vi "main.vi"() -> ()   [LabVIEW 2011]
uses:
  <vilib>/Simulation/Scripting/Companion Diagram/SimConfigNode/SimParams.ctl
  <vilib>/Simulation/Scripting/Companion Diagram/SimConfigNode/_simSolvers.ctl
  <vilib>/Simulation/Implementation/Shared/SIMSCR Execution Mode.ctl
  <vilib>/Simulation/Param Hierarchy/Typedefs/SIMPH Param Control Actions.ctl
  <vilib>/Simulation/Implementation/Shared/NILVSim_FinalizeModel.vi
  <vilib>/Simulation/Utility/Implementation/SIM Halt.vi
  <vilib>/Simulation/SignalDisplay/Implementation/NILVSim Time Waveform.llb/SIM Time Waveform (scalar).vi
  <vilib>/Simulation/DataSources/Implementation/NILVSim Step.llb/SIM Step (scalar).vi
  <vilib>/Simulation/DataSources/Implementation/NILVSim Pulse Generator.llb/SIM Pulse Generator (scalar).vi
  <vilib>/Simulation/DataSources/Implementation/NILVSim Ramp.llb/SIM Ramp (scalar).vi
  <vilib>/Simulation/DataSources/Implementation/NILVSim Sine Wave.llb/SIM Sine Wave (scalar).vi
  <vilib>/Simulation/DataSources/Implementation/NILVSim Chirp Signal.llb/SIM Chirp Signal (scalar).vi
  <vilib>/Simulation/ContinuousLinear/Implementation/NILVSim Transfer Function.llb/SIM Transfer Function Collector (SISO).vi
  <vilib>/Simulation/ContinuousLinear/Implementation/NILVSim Transfer Function.llb/SIM Transfer Function Distributor (SISO CD).vi
  <vilib>/Simulation/Implementation/Shared/SIM Is Init or Final Stage.vi
  <vilib>/Simulation/Implementation/Shared/NILVSim_Manager.vi
  <vilib>/Simulation/Implementation/Shared/NILVSim_ParamChanged.vi
  <vilib>/Simulation/Utility/Implementation/NILVSim Get Time and IsAcceptedStep.vi
  <vilib>/Simulation/Implementation/Shared/SIM Unbundle Sim Info.vi
  <vilib>/Simulation/Implementation/Shared/NILVSim_GetModelError.vi
  <vilib>/Simulation/Implementation/Shared/SIM Bundle Sim Info.vi
  <vilib>/Simulation/Implementation/Shared/NILVSim_Initialize.vi
  <vilib>/addons/Control Design/_Model Construction/Model Creation.llb/CD Construct Transfer Function Model.vi
  <vilib>/addons/Control Design/_Model Construction/Model Creation.llb/Model Creation SubVI/cd_Create Transfer Function Model.vi
  <vilib>/addons/Control Design/_Frequency Response Analysis/Frequency Response.llb/Frequency Response subVI/cd_Bode (Transfer Function).vi
  <vilib>/addons/Control Design/_Frequency Response Analysis/Frequency Response.llb/Frequency Response subVI/cd_Nyquist (Transfer Function).vi
  <vilib>/addons/Control Design/_Dynamic Analysis/Dynamic Analysis.llb/Dynamic Analysis subVI/cd_Root Locus (Transfer Function).vi
  <vilib>/Simulation/Scripting/Companion Diagram/SimConfigNode/SimDog.xnode
  <vilib>/Simulation/Implementation/XNodeFramework/SimXNode/SimX.xnode
  <vilib>/addons/Control Design/_Model Construction/NI_LinSys_Model Creation.lvlib
  <vilib>/addons/Control Design/_Model Construction/Model Typedefs.llb/CD General Elements.ctl
  <vilib>/addons/Control Design/_Model Construction/NI_LinSys_Model Typedefs.lvlib
  <vilib>/addons/Control Design/_Model Construction/Model Typedefs.llb/CD Transfer Function Model (SISO).ctl
  <vilib>/addons/Control Design/_Model Construction/Model Typedefs.llb/CD Transfer Function Model (MIMO).ctl
  <vilib>/Simulation/ContinuousLinear/Implementation/NILVSim Transfer Function.llb/SIM Transfer Function (SISO CD).vi
  <vilib>/addons/Control Design/_Frequency Response Analysis/NI_CD_Frequency Response.lvlib
  <vilib>/addons/Control Design/_Dynamic Analysis/NI_CD_Dynamic Analysis.lvlib
  <vilib>/Simulation/Implementation/Shared/NI_SIM_Implementation.lvlib
panel:
  in  "Tab In-Disp":enum32{""}(tab)
  out "Signal In":waveform(dbl)(graph)={"t0"=timestamp(9343.2 s since 1904-01-01), "dt"=1.0, "Y"=[0.2633720690985406]}
  in  "Halt Simulation":bool
  in  "Start Simulation":bool=TRUE
  in  "Tab In":enum32{"Step", "Ramp", "Pulse", "Sine", "Chirp"}(tab)
  in  "initial value":dbl
  in  "step time":dbl
  in  "final value":dbl=1.0
  in  "start time":dbl
  in  "slope":dbl=1.0
  in  "initial output":dbl
  in  "duty cycle":dbl=50.0
  in  "start time 2":dbl
  in  "period":dbl=2.0
  in  "amplitude":dbl=1.0
  in  "offset":dbl
  in  "offset 2":dbl
  in  "amplitude 2":dbl=1.0
  in  "frequency":dbl=0.5
  in  "phase":dbl
  in  "initial frequency":dbl=0.01
  in  "target time":dbl=10.0
  in  "target frequency":dbl=0.5
  in  "Tab Model":enum32{""}(tab)
  in  "Numerator":dbl[](array[numeric])=[1.0] format="%#.5g"
  in  "Denominator":dbl[](array[numeric])=[1.0, 1.0, 0.0, 0.0] format="%#.5g"
  in  "Delay":dbl format="%.2f"
  in  "Tab Out-Config":enum32{""}(tab)
  in  "Initial Time (s)":dbl
  in  "Final Time (s)":dbl=10.0
  in  "Tab Out-Display":enum32{""}(tab)
  out "Time Response":waveform(dbl)(graph)={"t0"=timestamp(10 s since 1904-01-01), "dt"=1.0, "Y"=[0.2054329974706435]}
  out "Bode Magnitude":cluster{"W":dbl[], "Magnitude":dbl[]}[](graph)
  out "Bode Phase":cluster{"W":dbl[], "Magnitude":dbl[]}[](graph)
  out "Root Locus Graph":cluster{dbl[], dbl[]}[](graph)=[{[], []}, {[-0.25, -0.25], [1.0897247358851685, -1.0897247358851685]}, {[], []}, {[], []}, {array[408 elements], array[408 elements]}, {array[408 elements], array[408 elements]}]
  out "Nyquist Plot":cluster{"W":dbl[], "Magnitude":dbl[]}[](graph)
  in  "Time Response":bool=TRUE
  in  "Bode":bool=TRUE
  in  "Nyquist":bool=TRUE
  in  "Root Locus":bool=TRUE
  in  "Out-Display":bool
  in  "Out-Simulation":bool
  in  "Model-Configure":bool
  in  "In-Config":bool
  in  "Type of signal":enum32{"Step", "Ramp", "Pulse", "Sine", "Chirp"}(radio)
  # "Signal In"
  # "Model"
  # "Signal Out"
  # "Signal In"
  # "Model"
  # "Signal Out"
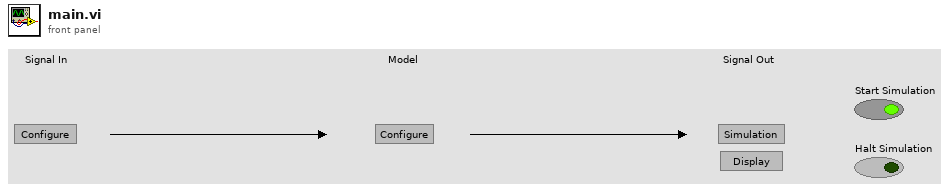
[diagram p1: front panel]
types:
  T1 = typedef "SIMPH Param Control Actions.ctl" = enum16{"get params", "set params"}
  T2 = typedef "SimParams.ctl" = cluster{"Initial Time (s)":dbl, "Final Time (s)":dbl, "Step Size (s)":dbl, "ODE Solver":T3, "Minimum Step Size (s)":dbl, "Maximum Step Size (s)":dbl, "Relative Tolerance":dbl, "Absolute Tolerance":dbl, "Software Timing":bool, "Initial Step Size (s)":dbl, "Automatic Fixed Step Size?":bool, "Automatic Discrete Step Size?":bool, "Discrete Step Size (s)":dbl, "Calculate using Time Step":bool, "Solver Wired?":bool, "Prev.Frm.Expected End":u64, "Prev.Frm.Actual End":u64, "Prev.Frm.Finished Late?":bool, "Prev.Iter.Expected End":u64, "Prev.Iter.Actual End":u64, "Prev.Iter.Finished Late?":bool, "Expected Iteration Start":u64, "Actual Iteration Start":u64, "Expected Frame Start":u64, "Actual Frame Start":u64, "Source Name":string, "Name":string, "Period":i64, "Deadline":i64, "Offset":i64, "Start":i64, "Priority":i32, "Timeout":i32, "Processor":i32, "Mode":enum32{"No Change", "Process missed periods, maintain original phase", "Discard missed periods, maintain original phase", "Process missed periods, ignore original phase", "Discard missed periods, ignore original phase"}, "Wakeup reason":enum32{"Normal", "Aborted", "Asynchronous wakeup", "Timing source error", "Timed loop error", "Timeout"}, "Error":errorcluster, "Source Type":string, "Secondary Source Type":string, "Global End Time":u64, "Global Start Time":u64, "Full Solver Reset":bool, "Execution Mode":T4, "Nan/Inf Check":bool, "Custom Solver Library":string, "Solver Is Variable":bool, "custom solver name":string}
  T3 = typedef "_simSolvers.ctl" = enum16{"Runge-Kutta 1 (Euler)", "Runge-Kutta 2", "Runge-Kutta 3", "Runge-Kutta 4", "Runge-Kutta 23 (variable)", "Runge-Kutta 45 (variable)", "BDF (variable)", "Adams-Moulton (variable)", "Rosenbrock (variable)", "Discrete States Only", "Linearizer", "State Query", "Trim Eval", "Custom Solver"}
  T4 = typedef "SIMSCR Execution Mode.ctl" = u16
  T5 = typedef "NI_LinSys_Model Typedefs.lvlib/CD Transfer Function Model (MIMO).ctl" = cluster{"properties":T6, "transfer function(s)":T7[][]}
  T6 = typedef "NI_LinSys_Model Typedefs.lvlib/CD General Elements.ctl" = cluster{"Model name":string, "Input names":string[], "Output names":string[], "Input Delays":dbl[], "Output Delays":dbl[], "Sampling Time":dbl, "Notes":string}
  T7 = typedef "NI_LinSys_Model Typedefs.lvlib/CD Transfer Function Model (SISO).ctl" = cluster{"Numerator":dbl[], "Denominator":dbl[], "delay":dbl}
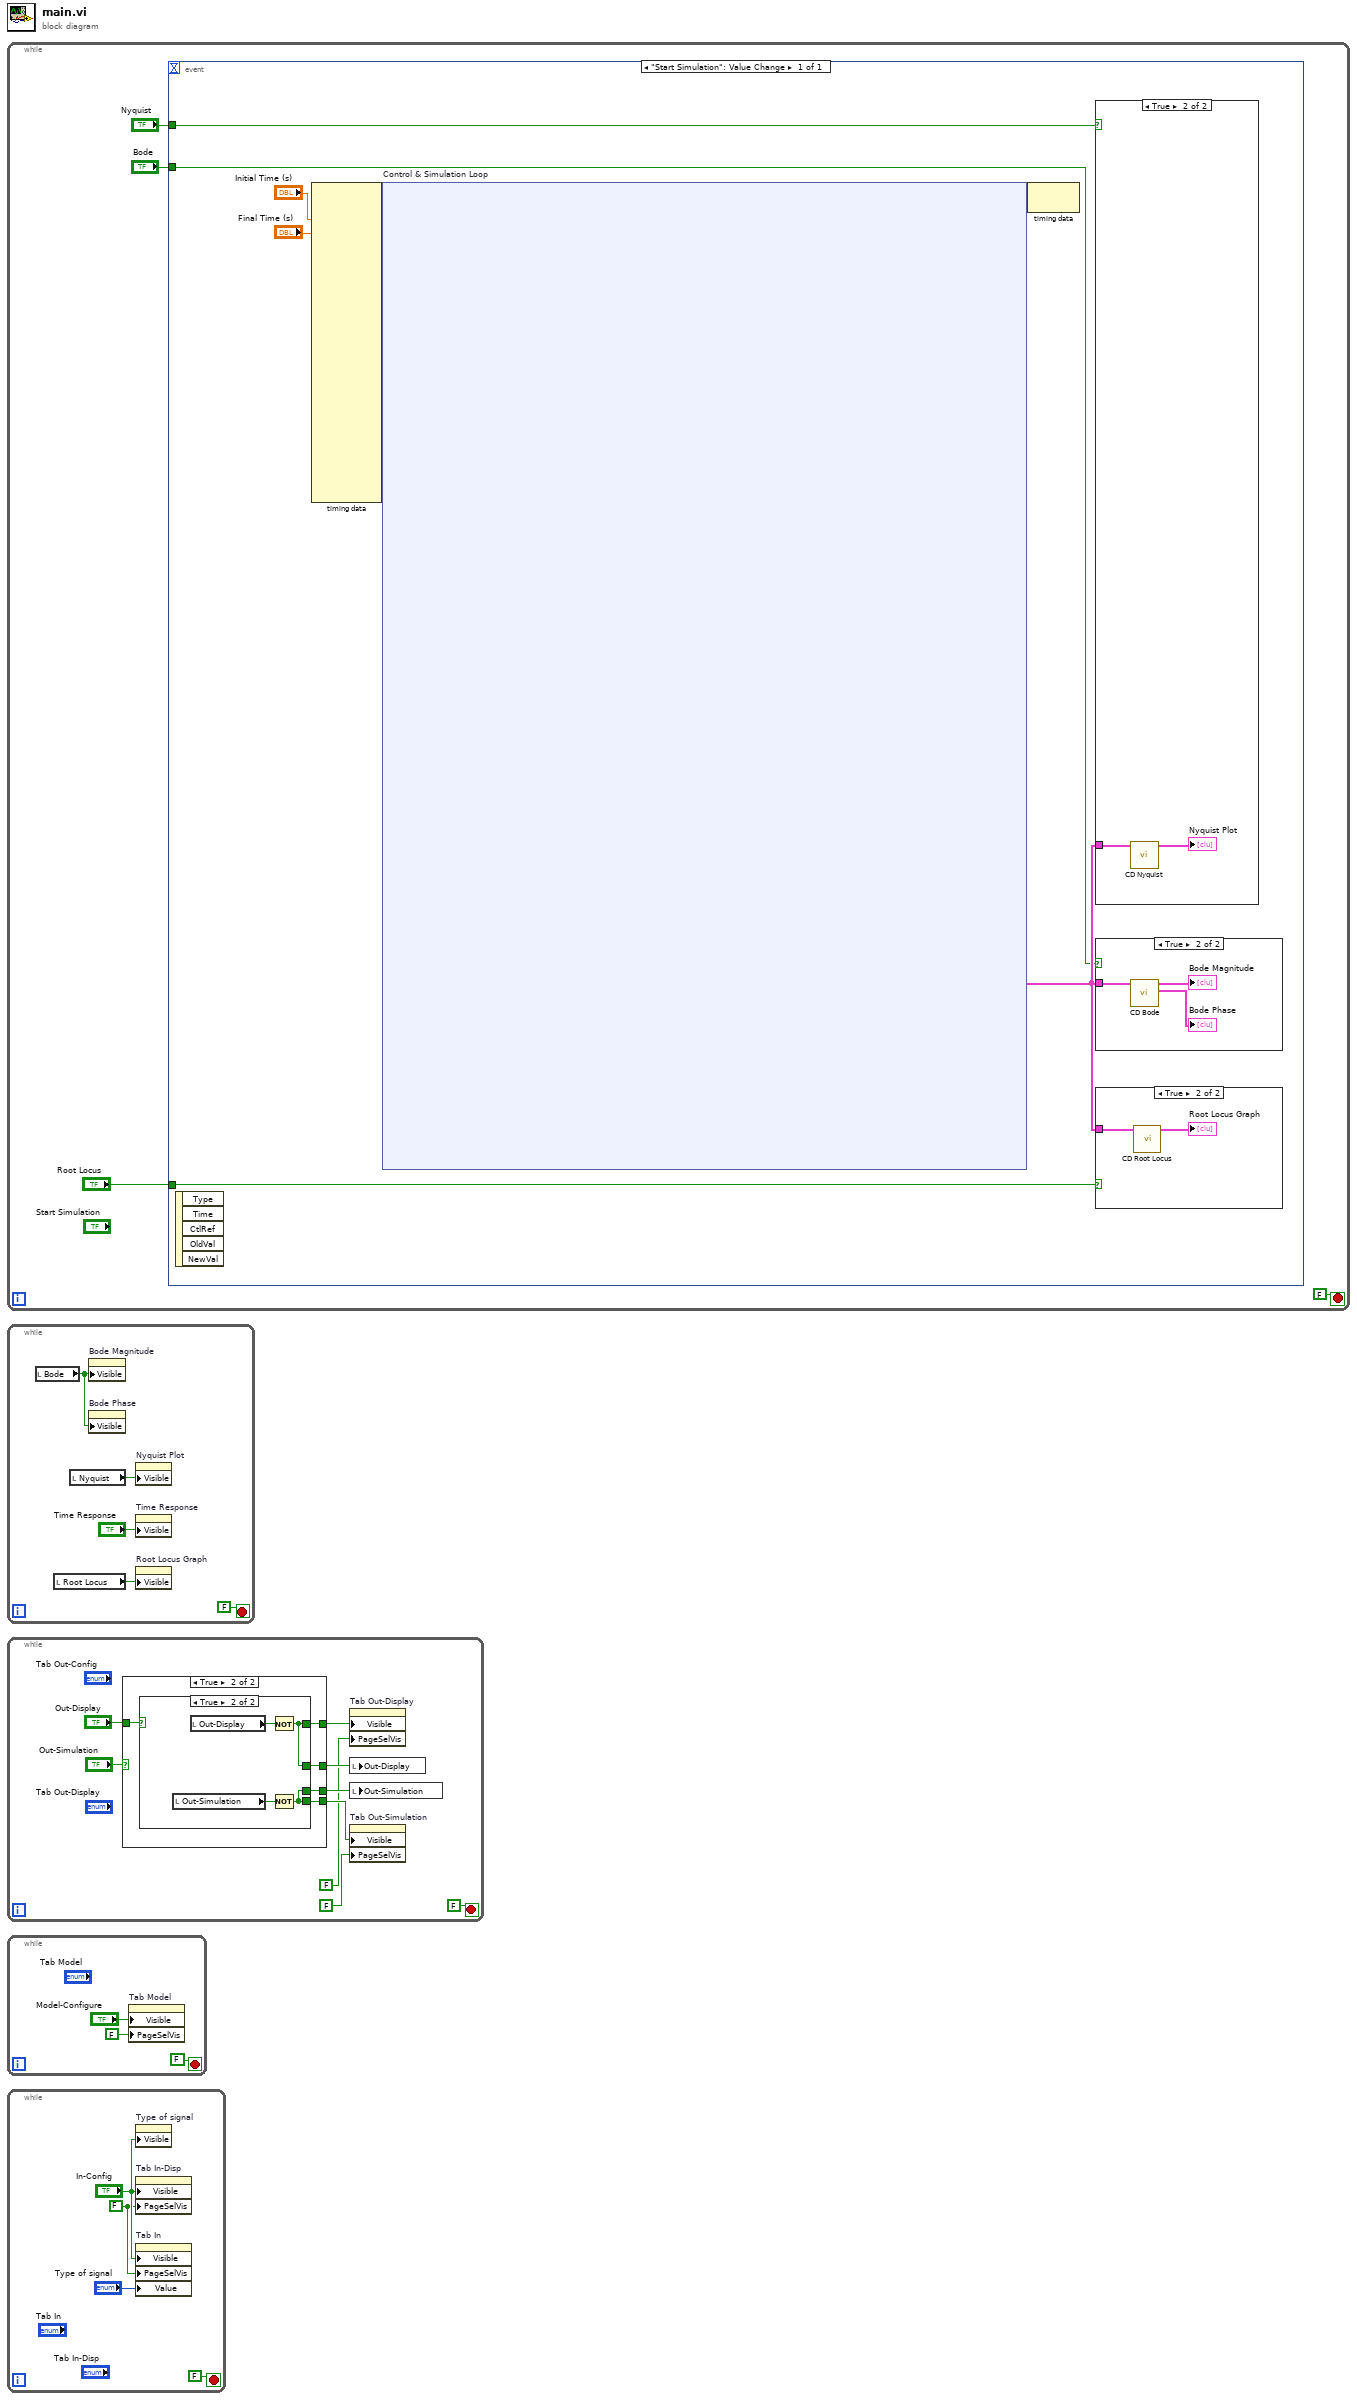
[diagram p0: block diagram]
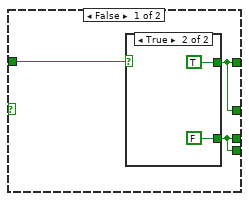
[diagram p2: hidden frame]
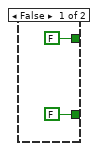
[diagram p3: hidden frame]
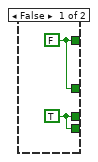
[diagram p4: hidden frame]
diagram:
  n1 = while {
    stop <- FALSE stop-if-true
    n2 = event shown="[0] \"Start Simulation\": Value Change" {
      selector: _ -> [_]
      dyn-events: _ -> [_]
      timeout: _ -> [_]
      tunnel: "Root Locus" -> [w7]
      tunnel: "Nyquist" -> [w6]
      tunnel: "Bode" -> [w5]
      event "Start Simulation": Value Change {
        n3 = event-data() -> ()  [unwired: 1 in, 5 out]
        n4 = node-c288("Initial Time (s)", "Final Time (s)") -> (w12:variant)  [unwired: 21 in]
        n5 = node-c254 "Control & Simulation Loop"(w12) -> (w11:variant, w8:T5)
        n6 = node-c288(w11) -> ()  [unwired: 1 out]
        n7 = case shown="True" w6 {
          tunnel: w8 -> [_ w13]
          frame False {
          }
          frame True {
            n8 = call-poly <vilib>:"CD Nyquist.vi"("Transfer Function Model"=w13) -> ("Nyquist Plot"=→"Nyquist Plot":cluster{"W":dbl[], "Magnitude":dbl[]}[])  [unwired: 8 in, 2 out]
          }
        }
        n9 = case shown="True" w5 {
          tunnel: w8 -> [_ w15]
          frame False {
          }
          frame True {
            n10 = call-poly <vilib>:"CD Bode.vi"("Transfer Function Model"=w15) -> ("Bode Phase"=→"Bode Phase":cluster{"W":dbl[], "Magnitude":dbl[]}[], "Bode Magnitude"=→"Bode Magnitude":cluster{"W":dbl[], "Magnitude":dbl[]}[])  [unwired: 6 in, 3 out]
          }
        }
        n11 = case shown="True" w7 {
          tunnel: w8 -> [_ w19]
          frame False {
          }
          frame True {
            n12 = call-poly <vilib>:"CD Root Locus.vi"("Transfer Function Model"=w19) -> ("Root Locus Graph"=→"Root Locus Graph":cluster{dbl[], dbl[]}[])  [unwired: 7 in, 3 out]
          }
        }
      }
    }
  }
  n13 = while {
    stop <- FALSE stop-if-true
    n14 = local read "Bode"() -> (w405:bool)
    n15 = local read "Root Locus"() -> (w404:bool)
    n16 = local read "Nyquist"() -> (w403:bool)
    n17 = property on="Bode Magnitude" class="XYGraph (strict)"("Visible"=w405) -> ()  [unwired: 2 in, 2 out]
    n18 = property on="Bode Phase" class="XYGraph (strict)"("Visible"=w405) -> ()  [unwired: 2 in, 2 out]
    n19 = property on="Nyquist Plot" class="XYGraph (strict)"("Visible"=w403) -> ()  [unwired: 2 in, 2 out]
    n20 = property on="Time Response" class="WFChart (strict)"("Visible"="Time Response") -> ()  [unwired: 2 in, 2 out]
    n21 = property on="Root Locus Graph" class="XYGraph (strict)"("Visible"=w404) -> ()  [unwired: 2 in, 2 out]
  }
  n22 = while {
    stop <- FALSE stop-if-true
    n23 = case shown="True" "Out-Simulation" {
      tunnel: "Out-Display" -> [w415 w426]
      tunnel: [w416 w425] -> w413
      tunnel: [w417 w424] -> w412
      tunnel: [w417 w423] -> w409
      tunnel: [w416 w422] -> w408
      frame False {
        n24 = case shown="True" w415 {
          tunnel: [FALSE ("Visible") FALSE ("Out-Simulation")] -> w416
          tunnel: [FALSE TRUE] -> w417
          frame False {
          }
          frame True {
          }
        }
      }
      frame True {
        n25 = case shown="True" w426 {
          tunnel: [w428 w432] -> w425
          tunnel: [w427 w429] -> w424
          tunnel: [w427 w429] -> w423
          tunnel: [w428 w432] -> w422
          frame False {
            w427 = FALSE
            w428 = TRUE ("Visible")
          }
          frame True {
            n26 = local read "Out-Simulation"() -> (w431:bool)
            n27 = local read "Out-Display"() -> (w430:bool)
            n28 = Not(x=w430) -> (.not. x?=w429:bool)
            n29 = Not(x=w431) -> (.not. x?=w432:bool)
          }
        }
      }
    }
    n30 = property on="Tab Out-Display" class="TabCtl (strict)"("Visible"=w412, "PageSelVis"=FALSE ("Page Selector Visible")) -> ()  [unwired: 2 in, 2 out]
    n31 = local write "Out-Display"(w409) -> ()
    n32 = local write "Out-Simulation"(w408) -> ()
    n33 = property on="Tab Out-Simulation" class="TabCtl (strict)"("Visible"=w413, "PageSelVis"=FALSE ("Page Selector Visible")) -> ()  [unwired: 2 in, 2 out]
  }
  n34 = while {
    stop <- FALSE stop-if-true
    n35 = property on="Tab Model" class="TabCtl (strict)"("Visible"="Model-Configure", "PageSelVis"=FALSE ("Page Selector Visible")) -> ()  [unwired: 2 in, 2 out]
  }
  n36 = while {
    stop <- FALSE stop-if-true
    w436 = FALSE ("Page Selector Visible")
    n37 = property on="Type of signal" class="RadioBtnsControl (strict)"("Visible"="In-Config") -> ()  [unwired: 2 in, 2 out]
    n38 = property on="Tab In-Disp" class="TabCtl (strict)"("Visible"="In-Config", "PageSelVis"=w436) -> ()  [unwired: 2 in, 2 out]
    n39 = property on="Tab In" class="TabCtl (strict)"("Visible"="In-Config", "PageSelVis"=w436, "Value"="Type of signal") -> ()  [unwired: 2 in, 2 out]
  }
